vi "ConfigureIncEncoderSensorType.vi"(4 "error in (no error)":errorcluster, 5 "incremental sensor type":u16(ring)=1 items=["Incremental encoder with index (3-channel)"=1, "Incremental encoder without index (2-channel)"=2], 6 "incremental encoder configuration":T1, 7 "axis in":cluster{"keyHandle":u32, "nodeId":u16}={"keyHandle"=0, "nodeId"=1}) -> (0 "error out":errorcluster, 3 "axis out":cluster{"keyHandle":u32, "nodeId":u16}={"keyHandle"=0, "nodeId"=1})   [LabVIEW 2018]
doc: "<B>ConfigureIncSensorType</B> writes the value for sensor type 'incremental encoder with index (3-channel)' to the device. Parameters from the sensor type can be set."
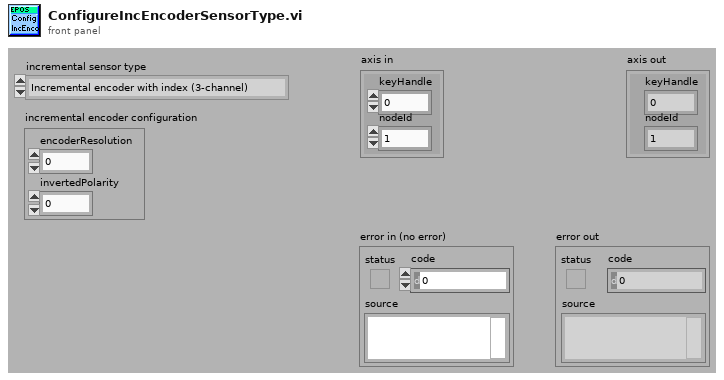
[diagram p1: front panel]
types:
  T1 = cluster{"encoderResolution":u32, "invertedPolarity":i32}
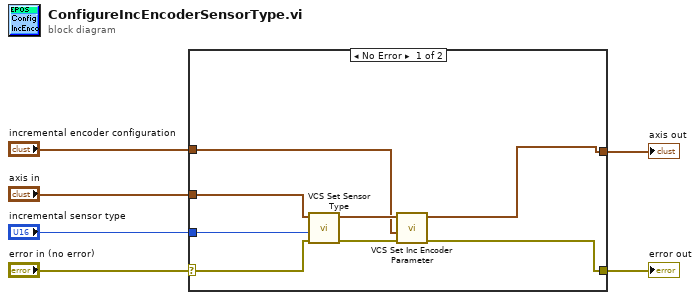
[diagram p0: block diagram]
diagram:
  n1 = case shown="No Error" "error in (no error)" {
    selector: "error in (no error)" -> [w13 w16]
    tunnel: [w7 w16] -> w5
    tunnel: [w8 w15] -> w4
    tunnel: "axis in" -> [w14 w15]
    tunnel: "incremental sensor type" -> [w12 _]
    tunnel: "incremental encoder configuration" -> [w9 _]
    frame No Error {
      n2 = call "VCS Set Sensor Type.vi"("error in (no error)"=w13, "SensorType"=w12, "axis in"=w14) -> ("error out"=w11:errorcluster, "axis out"=w10:cluster{"keyHandle":u32, "nodeId":u16})  [unwired: 7 in]
      n3 = call "VCS Set Inc Encoder Parameter.vi"("error in (no error)"=w11, "Incremental encoder"=w9, "axis in"=w10) -> ("error out"=w7:errorcluster, "axis out"=w8:cluster{"keyHandle":u32, "nodeId":u16})  [unwired: 7 in]
    }
    frame Error {
    }
  }
  "error out" <- w5
  "axis out" <- w4
